vi "NDHX Tube Wall Temperature.vi"(6 "Sec Temperature (K)":dbl, 9 "Air Temperature (K)":dbl, 10 "Air Heat Xfer Coeff":dbl, 11 "Sec Heat Xfer Coeff":dbl) -> (3 "Wall Temperature (K)":dbl)   [LabVIEW 2019]
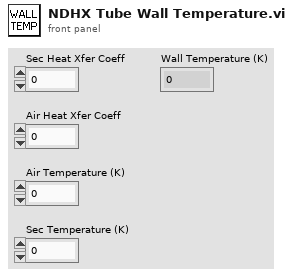
[diagram p1: front panel]
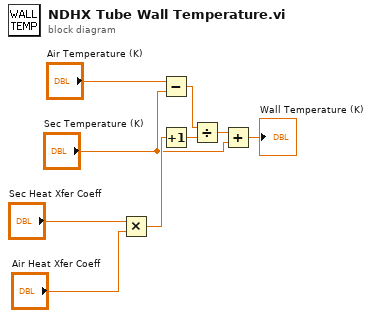
[diagram p0: block diagram]
diagram:
  n1 = Multiply(x="Sec Heat Xfer Coeff", y="Air Heat Xfer Coeff") -> (x*y=w8:dbl)
  n2 = Subtract(x="Air Temperature (K)", y="Sec Temperature (K)") -> (x-y=w3:dbl)
  n3 = Increment(x=w8) -> (x+1=w9:dbl)
  n4 = Divide(x=w3, y=w9) -> (x/y=w2:dbl)
  n5 = Add(x=w2, y="Sec Temperature (K)") -> (x+y=→"Wall Temperature (K)":dbl)
